vi "Q_Get Star Performers Events.vi"(8 "error in (no error)":errorcluster, 11 "Data Manager in":refnum<class "Data Manager.lvclass">) -> (0 "error out":errorcluster, 2 "All Tables":T1(array[cluster]), 3 "Data Manager out":refnum<class "Data Manager.lvclass">)   [LabVIEW 2020, in "Data Manager.lvclass"]
uses:
  Data Manager.lvclass
  Data Manager.lvclass/Data Manager.ctl
  <vilib>/drjdpowell/SQLite Library/SQL Connection/Execute SQL.vi
  <vilib>/drjdpowell/SQLite Library/SQLite.lvlib
  <vilib>/drjdpowell/SQLite Library/SQL Connection/Connection.lvclass
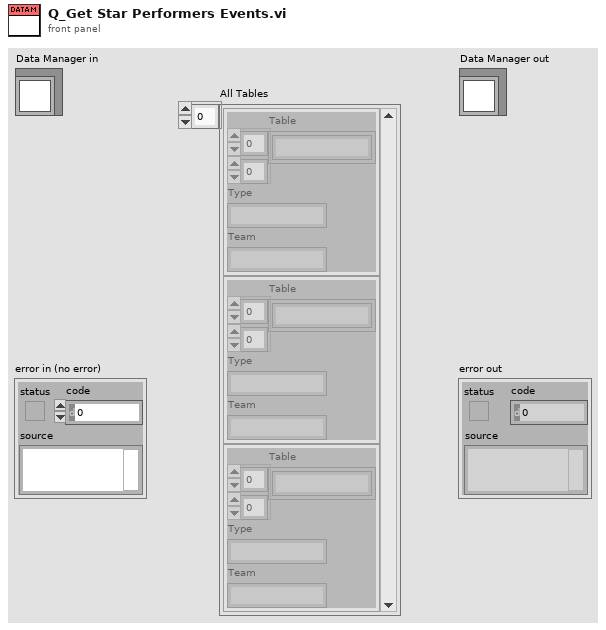
[diagram p1: front panel]
types:
  T1 = cluster{"Table":string[][], "Type":string, "Team":string}[]
  T2 = cluster{"Table":string[][], "Type":string, "Team":string}
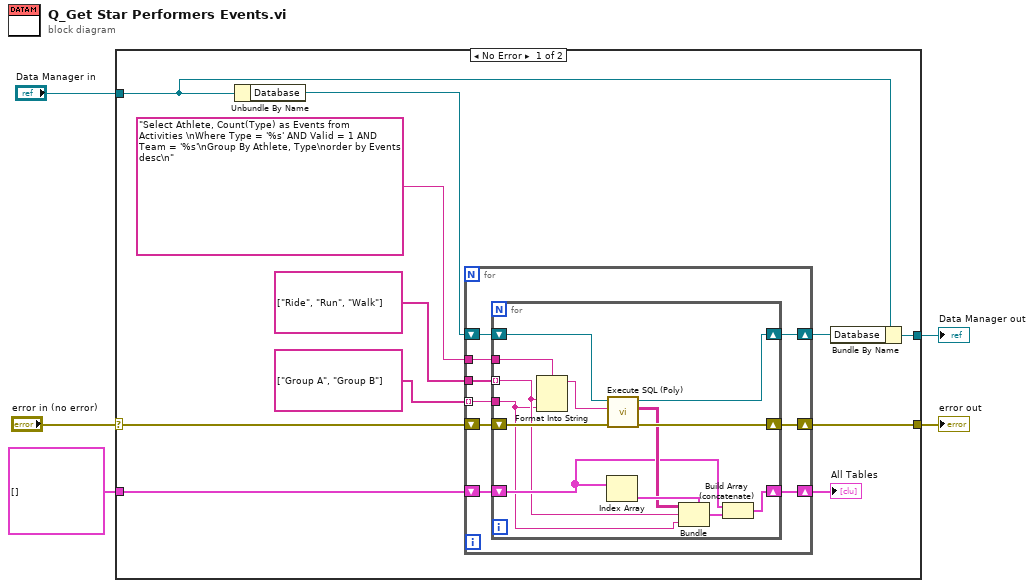
[diagram p0: block diagram]
diagram:
  n1 = case shown="No Error" "error in (no error)" {
    selector: "error in (no error)" -> [w12 w40]
    tunnel: [w11 w40] -> w4
    tunnel: [w14 w39] -> w2
    tunnel: "Data Manager in" -> [w15 w39]
    tunnel: T1 [] ("All Tables") -> [w7 _]
    frame No Error {
      n2 = Unbundle By Name(w15) -> ("Database"=w16:refnum<class "Connection.lvclass">)
      n3 = for {
        tunnel: "Select Athlete, Count(Type) as Events from Activities \nWhere Type = '%s' AND Valid = 1 AND Team = '%s'\nGroup By Athlete, Type\norder by Events desc\n" ("SQL") -> [w21]
        shift-right: [w24] -> w13
        shift-left: w16 -> [w25]
        shift-right: [w22] -> w11
        shift-left: w12 -> [w23]
        tunnel: string[] ["Ride", "Run", "Walk"] -> [w20]
        tunnel: string[] ["Group A", "Group B"] -> [w19] mode=indexing
        shift-right: [w17] -> w6
        shift-left: w7 -> [w18]
        n4 = for {
          tunnel: w21 -> [w34]
          shift-right: [w37] -> w24
          shift-left: w25 -> [w38]
          shift-right: [w35] -> w22
          shift-left: w23 -> [w36]
          tunnel: w20 -> [w27] mode=indexing
          tunnel: w19 -> [w26]
          shift-right: [w29] -> w17
          shift-left: w18 -> [w28]
          n5 = Format Into String(format string=w34, w27, w26) -> (resulting string=w33:string)  [unwired: 2 in, 1 out]
          n6 = Index Array(array=w28) -> (element=w32:T2)  [unwired: 1 in]
          n7 = call-poly <vilib>:"Execute SQL (Poly).vi"("error in (no error)"=w36, "SQL"=w33, "SQLite Connection in"=w38) -> ("error out"=w35:errorcluster, "Result Set"=w31:string[][], "SQLite Connection"=w37:refnum<class "Connection.lvclass">)  [unwired: 5 in, 1 out]
          n8 = Bundle(cluster=w32, "Table"=w31, "Type"=w27, "Team"=w26) -> (w30:T2)
          n9 = Build Array (concatenate)(w28, w30) -> (w29:T1)
        }
      }
      "All Tables" <- w6
      n10 = Bundle By Name(cluster=w15, "Database"=w13) -> (w14:refnum<class "Data Manager.lvclass">)
    }
    frame Error {
    }
  }
  "error out" <- w4
  "Data Manager out" <- w2
